vi "SeCrTs-Stop Read FGV.vi"(7 "Enum":enum16{"Init", "Read", "Write"}(ring), 11 "Stop":bool) -> (3 "Stop R":bool)   [LabVIEW 2022 SP3]
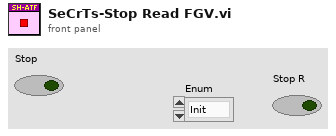
[diagram p1: front panel]
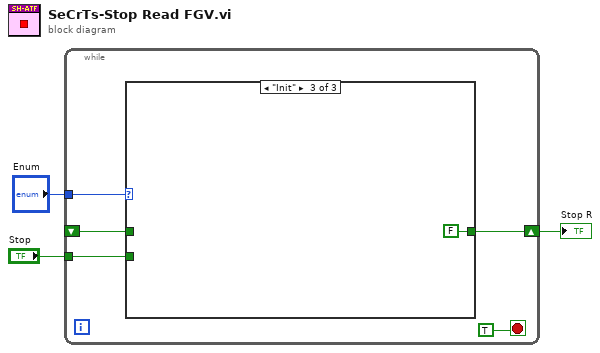
[diagram p0: block diagram]
diagram:
  n1 = while {
    tunnel: "Enum" -> [w8]
    tunnel: "Stop" -> [w6]
    shift-right: [w5] -> w1
    shift-left: _ -> [w4]
    stop <- TRUE stop-if-true
    n2 = case shown="\"Init\"" w8 {
      tunnel: w6 -> [_ w10 _]
      tunnel: [w9 w10 FALSE ("Exit")] -> w5
      tunnel: w4 -> [w9 _ _]
      frame "Read", Default {
      }
      frame "Write" {
      }
      frame "Init" {
      }
    }
  }
  "Stop R" <- w1
